vi "main.vi"() -> ()   [LabVIEW 2019]
uses:
  typedefs/basic_configuration_cluster.ctl
  typedefs/test_configuration_cluster.ctl
  typedefs/states.ctl
  typedefs/converter_configuration_cluster.ctl
  typedefs/log_data_cluster.ctl
  typedefs/operation.ctl
  typedefs/command.ctl
  <vilib>/Instr/_visa.llb/VISA Configure Serial Port (Instr).vi
panel:
  out "Configuration":T1(tab)
  in  "Ready":bool
  in  "Virtual COM port":refnum<visa-resource-name>="COM12"
  in  "Write":bool
  in  "Read":bool
  in  "data to write":T2={"version"=1, "const. voltage (mV)"=4200, "end-of-postdischarge (mAh)"=1750, "end-of-discharge (mV)"=2500, "end-of-precharge (mA or mV)"=100, "end-of-charge (mA or mV)"=100, "capacity (mAh)"=3500, "const. current char (mA)"=1750, "const. current disc (mA)"=3500} {"version" items=["Li-Ion"=1, "Ni-MH"=2]}
  out "received data":T2={"version"=1, "const. voltage (mV)"=0, "end-of-postdischarge (mAh)"=1750, "end-of-discharge (mV)"=2500, "end-of-precharge (mA or mV)"=100, "end-of-charge (mA or mV)"=100, "capacity (mAh)"=3500, "const. current char (mA)"=3500, "const. current disc (mA)"=0} {"version" items=["Li-Ion"=1, "Ni-MH"=2]}
  out "Sent":string
  out "Received":string
  out "Reception errors":string
  in  "to converter configuration":bool
  out "received data":T3={"number of cells"=1, "number of states "=8, "number of repetitions"=1, "end wait time (s)"=1200, "wait time (s)"=600, "1st state"=5, "2nd state"=11, "3rd state"=7, "4th state"=11, "5th state"=3, "6th state"=11, "7th state"=9, "8th state"=11, "9th state"=0, "10th state"=0} {"10th state" items=["not defined"=0, "charge"=3, "precharge"=5, "discharge"=7, "postdischarge"=9, "DC Resistance"=11]; "9th state" items=["not defined"=0, "charge"=3, "precharge"=5, "discharge"=7, "postdischarge"=9, "DC Resistance"=11]; "8th state" items=["not defined"=0, "charge"=3, "precharge"=5, "discharge"=7, "postdischarge"=9, "DC Resistance"=11]; "7th state" items=["not defined"=0, "charge"=3, "precharge"=5, "discharge"=7, "postdischarge"=9, "DC Resistance"=11]; "6th state" items=["not defined"=0, "charge"=3, "precharge"=5, "discharge"=7, "postdischarge"=9, "DC Resistance"=11]; "5th state" items=["not defined"=0, "charge"=3, "precharge"=5, "discharge"=7, "postdischarge"=9, "DC Resistance"=11]; "4th state" items=["not defined"=0, "charge"=3, "precharge"=5, "discharge"=7, "postdischarge"=9, "DC Resistance"=11]; "3rd state" items=["not defined"=0, "charge"=3, "precharge"=5, "discharge"=7, "postdischarge"=9, "DC Resistance"=11]; "2nd state" items=["not defined"=0, "charge"=3, "precharge"=5, "discharge"=7, "postdischarge"=9, "DC Resistance"=11]; "1st state" items=["not defined"=0, "charge"=3, "precharge"=5, "discharge"=7, "postdischarge"=9, "DC Resistance"=11]}
  out "Reception errors":string
  in  "Read 2":bool
  in  "Write 2":bool
  out "Sent":string
  out "Received":string
  in  "to test":bool
  in  "data to write":T3={"number of cells"=1, "number of states "=8, "number of repetitions"=1, "end wait time (s)"=1200, "wait time (s)"=600, "1st state"=5, "2nd state"=11, "3rd state"=7, "4th state"=11, "5th state"=3, "6th state"=11, "7th state"=9, "8th state"=11, "9th state"=0, "10th state"=0} {"10th state" items=["not defined"=0, "charge"=3, "precharge"=5, "discharge"=7, "postdischarge"=9, "DC Resistance"=11]; "9th state" items=["not defined"=0, "charge"=3, "precharge"=5, "discharge"=7, "postdischarge"=9, "DC Resistance"=11]; "8th state" items=["not defined"=0, "charge"=3, "precharge"=5, "discharge"=7, "postdischarge"=9, "DC Resistance"=11]; "7th state" items=["not defined"=0, "charge"=3, "precharge"=5, "discharge"=7, "postdischarge"=9, "DC Resistance"=11]; "6th state" items=["not defined"=0, "charge"=3, "precharge"=5, "discharge"=7, "postdischarge"=9, "DC Resistance"=11]; "5th state" items=["not defined"=0, "charge"=3, "precharge"=5, "discharge"=7, "postdischarge"=9, "DC Resistance"=11]; "4th state" items=["not defined"=0, "charge"=3, "precharge"=5, "discharge"=7, "postdischarge"=9, "DC Resistance"=11]; "3rd state" items=["not defined"=0, "charge"=3, "precharge"=5, "discharge"=7, "postdischarge"=9, "DC Resistance"=11]; "2nd state" items=["not defined"=0, "charge"=3, "precharge"=5, "discharge"=7, "postdischarge"=9, "DC Resistance"=11]; "1st state" items=["not defined"=0, "charge"=3, "precharge"=5, "discharge"=7, "postdischarge"=9, "DC Resistance"=11]}
  in  "converter configuration cluster":T5={"CVKp (x1E-3)"=1, "CVKi (x1E-3)"=8, "CVKd (x1E-1)"=1, "CCKi (x1E-3)"=1200, "CCKp (x1E-3)"=600}
  in  "Write 3":bool
  in  "Read 3":bool
  in  "to test 2":bool
  out "Received":string
  out "Sent":string
  out "Reception errors":string
  out "received data":T5={"CVKp (x1E-3)"=1, "CVKi (x1E-3)"=8, "CVKd (x1E-1)"=1, "CCKi (x1E-3)"=1200, "CCKp (x1E-3)"=600}
  out "Temperature":T6(graph)
  out "Test graph":T7(graph)
  in  "reset":bool
  in  "start":bool
  in  "next cell":bool
  in  "next state":bool
  out "log data cluster":T8={"cell counter"=1, "repetition counter"=8, "state"=1, "elapsed time (s)"=600, "voltage (mV)"=1200, "current (mA)"=1200, "capacity (mAh)"=1200, "temperature (x10E-2°C)"=1200, "duty cycle (x10E-3)"=1200}
  out "tests":bool
  out "current state":T4=1 items=["not defined"=0, "stand by"=1, "charge"=3, "precharge"=5, "discharge"=7, "postdischarge"=9, "DC Resistance"=11, "wait"=13]
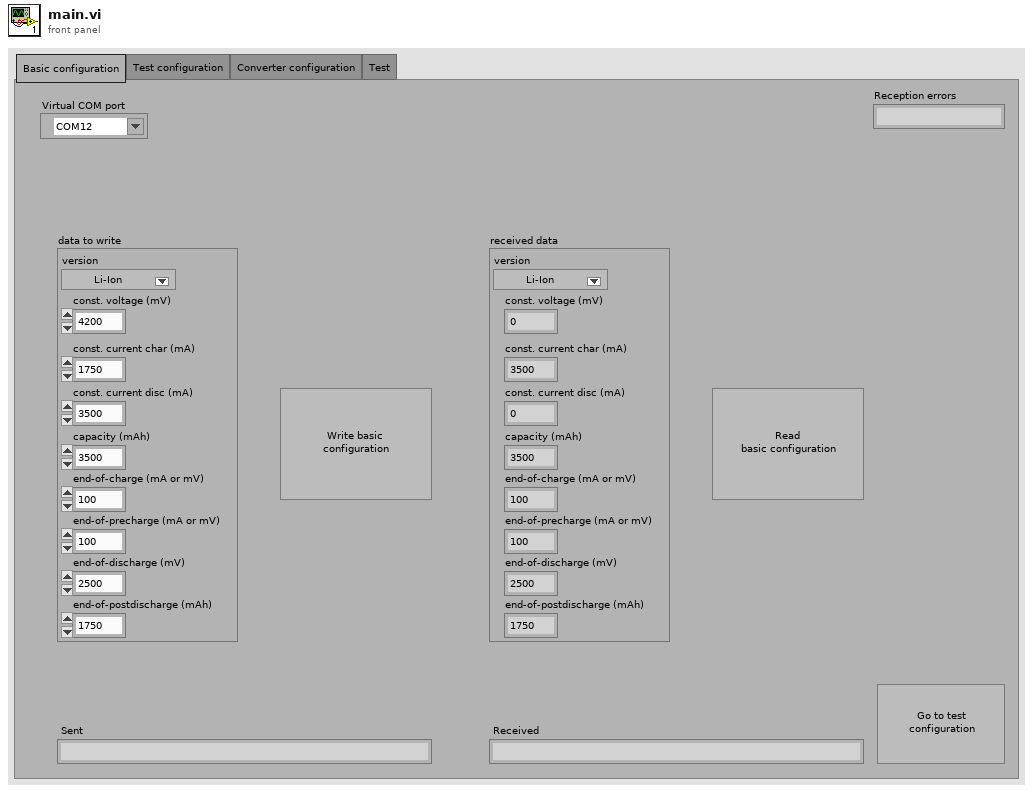
[diagram p1: front panel]
types:
  T1 = enum32{"Basic configuration", "Test configuration", "Converter configuration", "Test"}
  T2 = typedef "basic_configuration_cluster.ctl" = cluster{"version":u8, "const. voltage (mV)":u16, "end-of-postdischarge (mAh)":u16, "end-of-discharge (mV)":u16, "end-of-precharge (mA or mV)":u16, "end-of-charge (mA or mV)":u16, "capacity (mAh)":u16, "const. current char (mA)":u16, "const. current disc (mA)":u16}
  T3 = typedef "test_configuration_cluster.ctl" = cluster{"number of cells":u8, "number of states ":u8, "number of repetitions":u8, "end wait time (s)":u16, "wait time (s)":u16, "1st state":T4, "2nd state":T4, "3rd state":T4, "4th state":T4, "5th state":T4, "6th state":T4, "7th state":T4, "8th state":T4, "9th state":T4, "10th state":T4}
  T4 = typedef "states.ctl" = u8
  T5 = typedef "converter_configuration_cluster.ctl" = cluster{"CVKp (x1E-3)":u16, "CVKi (x1E-3)":u16, "CVKd (x1E-1)":u16, "CCKi (x1E-3)":u16, "CCKp (x1E-3)":u16}
  T6 = cluster{"elapsed time (s)":u16, "voltage (mV)":u16}[]
  T7 = cluster{cluster{"elapsed time (s)":u16, "capacity (mAh)":u16}[]}[]
  T8 = typedef "log_data_cluster.ctl" = cluster{"cell counter":u8, "repetition counter":u8, "state":u8, "elapsed time (s)":u16, "voltage (mV)":u16, "current (mA)":u16, "capacity (mAh)":u16, "temperature (x10E-2°C)":u16, "duty cycle (x10E-3)":u16}
  T9 = typedef "operation.ctl" = enum16{"wait", "read", "write", "action"}
  T10 = enum16{"big-endian, network order", "native, host order", "little-endian"}
  T11 = typedef "command.ctl" = enum16{"basic configuration", "test configuration", "converter configuration", "reset", "start", "next cell", "next state"}
  T12 = cluster{"elapsed time (s)":u16, "temperature (x10E-2°C)":u16}
  T13 = cluster{"elapsed time (s)":u16, "current (mA)":u16}
  T14 = cluster{"elapsed time (s)":u16, "capacity (mAh)":u16}
  T15 = cluster{"elapsed time (s)":u16, "voltage (mV)":u16}
  T16 = cluster{cluster{"elapsed time (s)":u16, "voltage (mV)":u16}[]}
  T17 = cluster{cluster{"elapsed time (s)":u16, "voltage (mV)":u16}[]}[]
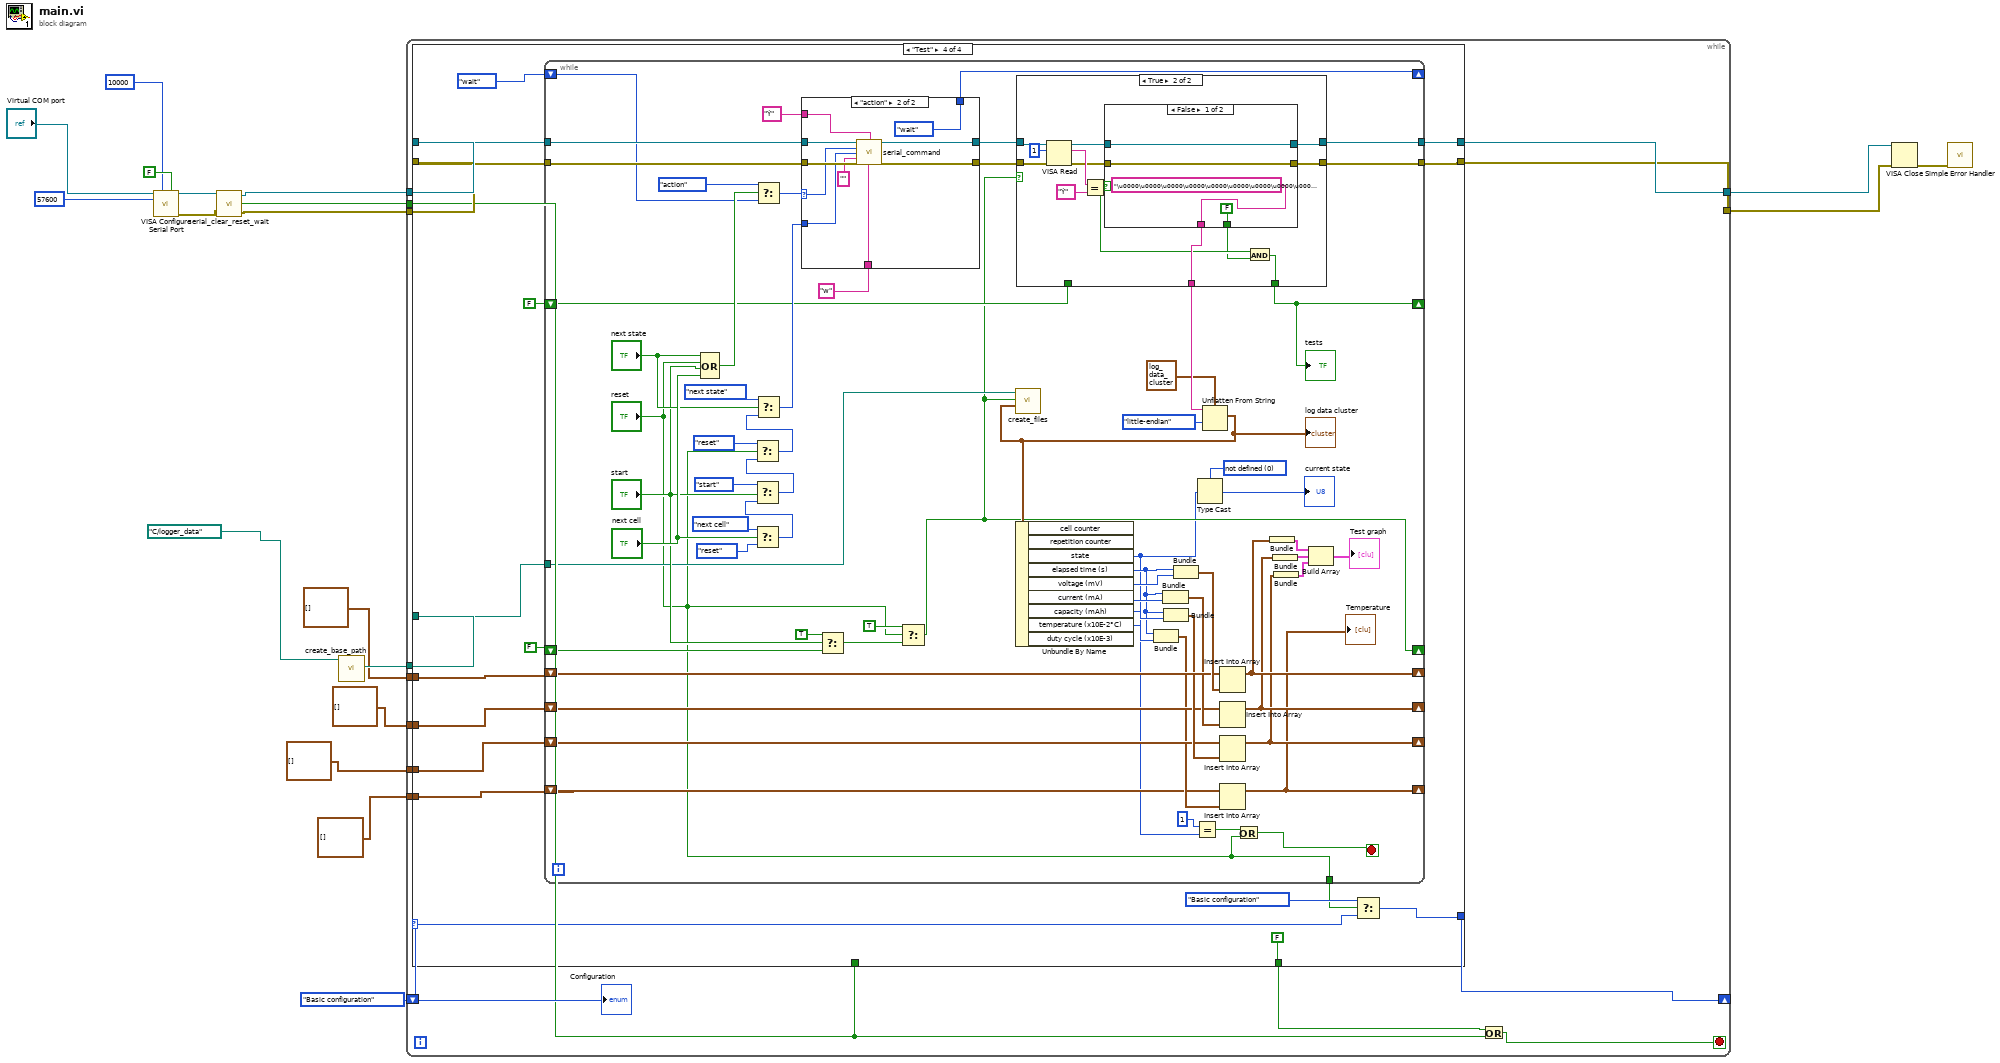
[diagram p0: block diagram]
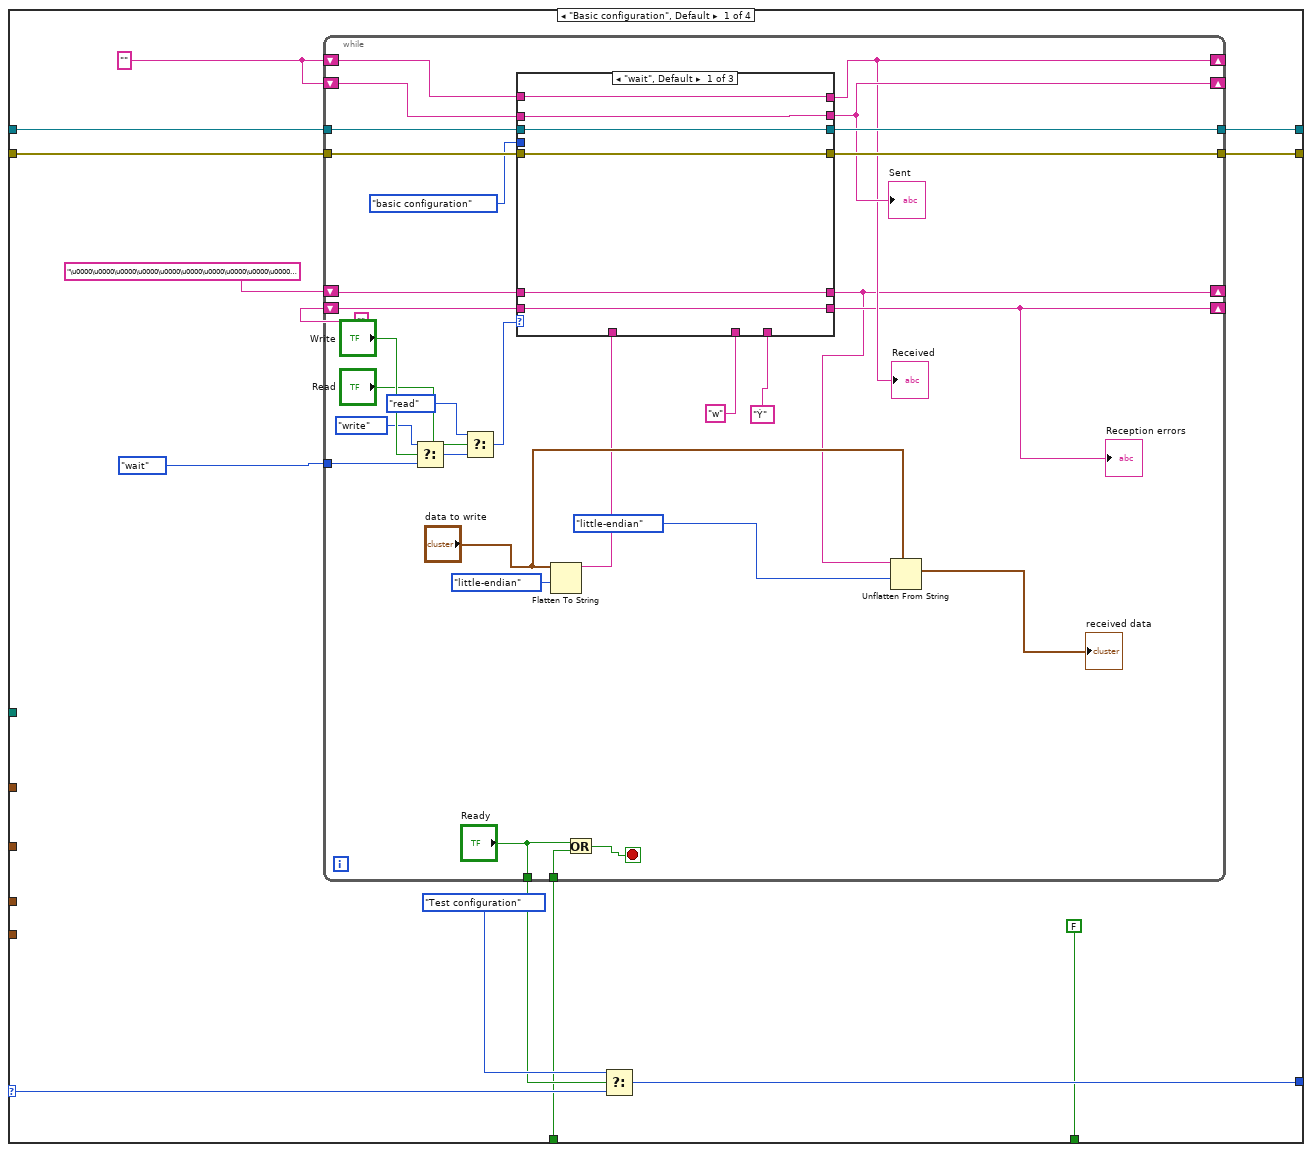
[diagram p2: hidden frame]
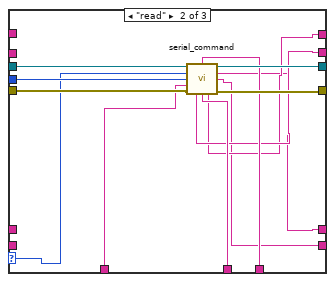
[diagram p3: hidden frame]
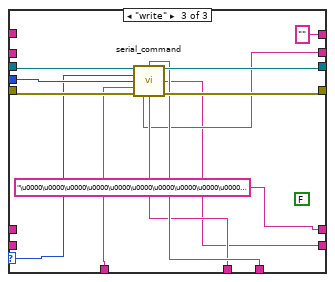
[diagram p4: hidden frame]
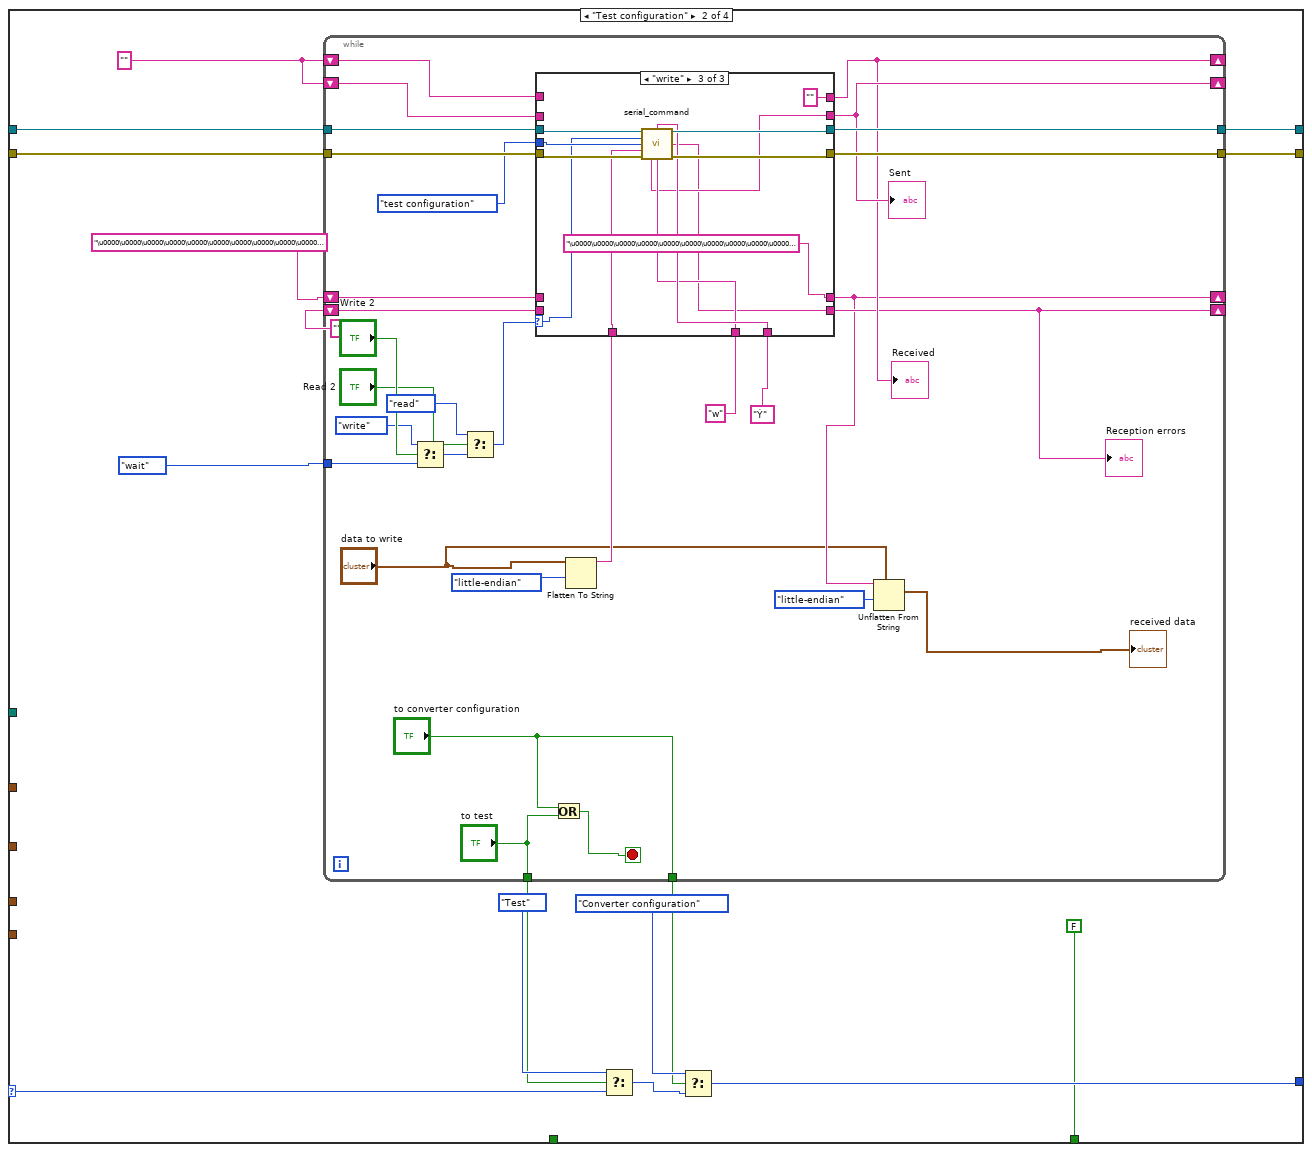
[diagram p5: hidden frame]
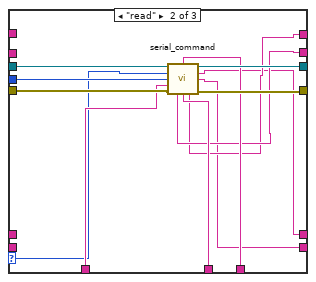
[diagram p7: hidden frame]
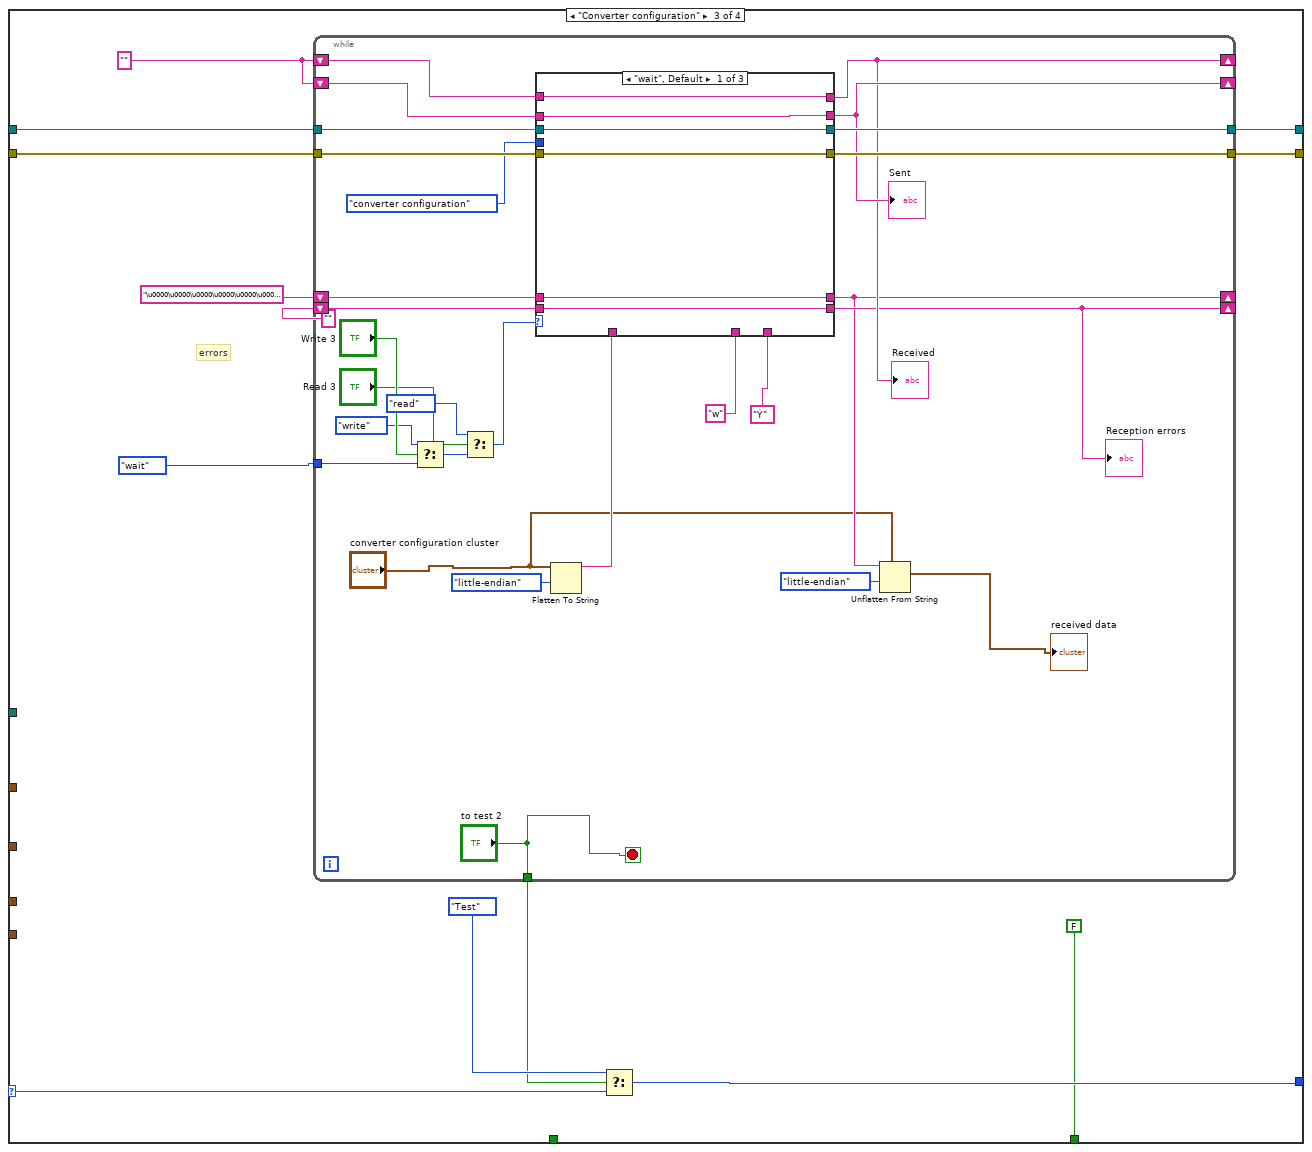
[diagram p8: hidden frame]
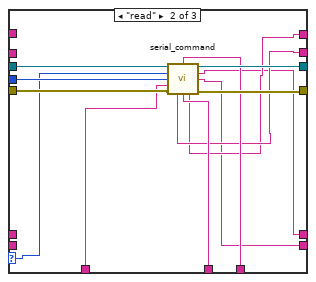
[diagram p9: hidden frame]
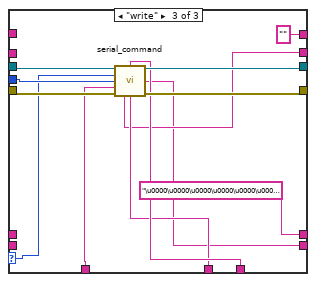
[diagram p10: hidden frame]
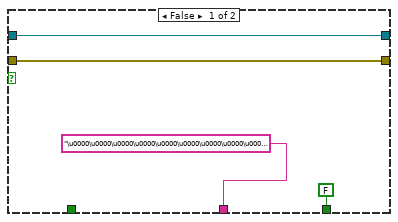
[diagram p11: hidden frame]
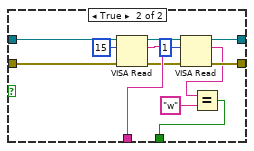
[diagram p12: hidden frame]
diagram:
  n1 = call-poly "VISA Configure Serial Port"("VISA resource name"="Virtual COM port", "timeout (10sec)"=u32 10000, "Enable Termination\nChar (T)"=FALSE ("Enable Termination\nChar (T)"), "baud rate (9600)"=u32 57600) -> ("VISA resource name out"=w17:refnum<visa-resource-name>, "error out"=w16:errorcluster)  [unwired: 10 in]
  n2 = call "serial_clear_reset_wait.vi"("VISA Refnum in"=w17, "error in (no error)"=w16) -> ("VISA Refnum out"=w12:refnum<visa-resource-name>, "test"=w8:bool, "error out"=w11:errorcluster)
  n3 = call "create_base_path.vi"("folder"=path "C:/logger_data") -> ("appended path"=w10:path)  [unwired: 10 in]
  n4 = while {
    shift-right: [w33] -> _
    shift-left: T1."Basic configuration" ("Configuration") -> [w29]
    tunnel: w12 -> [w32]
    tunnel: w11 -> [w26]
    tunnel: [w31] -> w7
    tunnel: [w30] -> w6
    tunnel: w10 -> [w28]
    tunnel: w8 -> [w25]
    tunnel: T6 [] -> [w24]
    tunnel: T6 [] -> [w23]
    tunnel: T6 [] -> [w22]
    tunnel: T6 [] -> [w21]
    stop <- w27 stop-if-true
    n5 = case shown="\"Test\"" w29 {
      selector: w29 -> [w47 w125 w200 w262]
      tunnel: [w46 w113 w191 w261] -> w33
      tunnel: w32 -> [w43 w122 w197 w276]
      tunnel: w26 -> [w42 w121 w196 w275]
      tunnel: [w41 w120 w195 w274] -> w31
      tunnel: [w40 w119 w194 w273] -> w30
      tunnel: [FALSE ("reset") FALSE ("reset") FALSE ("reset") FALSE ("reset")] -> w20
      tunnel: w28 -> [_ _ _ w270]
      tunnel: w25 -> [w34 _ _ _]
      tunnel: w24 -> [_ _ _ w269]
      tunnel: w23 -> [_ _ _ w268]
      tunnel: w22 -> [_ _ _ w267]
      tunnel: w21 -> [_ _ _ w266]
      frame "Basic configuration", Default {
        w38 = ""
        n6 = while {
          tunnel: ["Ready"] -> w44
          tunnel: w43 -> [w77]
          tunnel: w42 -> [w75]
          tunnel: [w76] -> w41
          tunnel: [w74] -> w40
          tunnel: operation."wait" -> [w73]
          shift-right: [w66] -> _
          shift-left: w38 -> [w65]
          shift-right: [w60] -> _
          shift-left: w38 -> [w64]
          shift-right: [w58] -> _
          shift-left: "" -> [w59]
          shift-right: [w53] -> _
          shift-left: "\u0000\u0000\u0000\u0000\u0000\u0000\u0000\u0000\u0000\u0000\u0000\u0000\u0000\u0000\u0000\u0000\u0000" ("data string") -> [w51]
          tunnel: w34 -> [w48]
          stop <- w50 stop-if-true
          n7 = Select(t=operation."write", s="Write", f=w73) -> (s? t:f=w70:T9)
          n8 = Select(t=operation."read", s="Read", f=w70) -> (s? t:f=w69:T9)
          n9 = Flatten To String(anything="data to write", byte order (0:big-endian, network order)=T10."little-endian") -> (data string=w52:string)  [unwired: 2 in, 2 out]
          n10 = case shown="\"wait\", Default" w69 {
            selector: w69 -> [_ w86 w99]
            tunnel: w77 -> [w83 w96 w109]
            tunnel: [w83 w94 w106] -> w76
            tunnel: w75 -> [w82 w95 w108]
            tunnel: [w82 w93 w105] -> w74
            tunnel: [w81 w90 w101] -> w66
            tunnel: w65 -> [w81 _ _]
            tunnel: [w80 w89 "" ("disassembled command")] -> w60
            tunnel: w64 -> [w80 _ _]
            tunnel: w52 -> [_ w87 w102]
            tunnel: "w" ("stop byte") -> [_ w92 w103]
            tunnel: "Ý" ("start byte") -> [_ w91 w104]
            tunnel: command."basic configuration" ("command code enum") -> [_ w88 w107]
            tunnel: w59 -> [w79 _ _]
            tunnel: [w79 w85 w97] -> w58
            tunnel: w51 -> [w78 _ _]
            tunnel: [w78 w84 "\u0000\u0000\u0000\u0000\u0000\u0000\u0000\u0000\u0000\u0000\u0000\u0000\u0000\u0000\u0000\u0000\u0000" ("data string")] -> w53
            frame "wait", Default {
            }
            frame "read" {
              n11 = call "serial_command.vi"("VISA in"=w96, "start byte"=w91, "operation enum"=w86, "command code enum"=w88, "data"=w87, "error in"=w95, "stop byte"=w92) -> ("VISA out"=w94:refnum<visa-resource-name>, "data"=w84:string, "error"=w85:string, "assembled command"=w90:string, "disassembled command"=w89:string, "error out"=w93:errorcluster)  [unwired: 1 in, 2 out]
            }
            frame "write" {
              (unwired) FALSE ("tests")
              n12 = call "serial_command.vi"("VISA in"=w109, "start byte"=w104, "operation enum"=w99, "command code enum"=w107, "data"=w102, "error in"=w108, "stop byte"=w103) -> ("VISA out"=w106:refnum<visa-resource-name>, "error"=w97:string, "assembled command"=w101:string, "error out"=w105:errorcluster)  [unwired: 1 in, 4 out]
            }
          }
          "Sent" <- w66
          "Received" <- w60
          "Reception errors" <- w58
          n13 = Or(x="Ready", y=w48) -> (x .or. y?=w50:bool)
          n14 = Unflatten From String(type="data to write", binary string=w53, byte order (0:big-endian, network order)=T10."little-endian") -> (value=→"received data":T2)  [unwired: 2 in, 2 out]
        }
        n15 = Select(t=T1."Test configuration", s=w44, f=w47) -> (s? t:f=w46:T1)
      }
      frame "Test configuration" {
        w117 = ""
        n16 = while {
          tunnel: ["to test"] -> w123
          tunnel: w122 -> [w155]
          tunnel: w121 -> [w153]
          tunnel: [w154] -> w120
          tunnel: [w152] -> w119
          tunnel: operation."wait" -> [w151]
          shift-right: [w144] -> _
          shift-left: w117 -> [w143]
          shift-right: [w137] -> _
          shift-left: w117 -> [w142]
          tunnel: ["to converter configuration"] -> w114
          shift-right: [w132] -> _
          shift-left: "" -> [w133]
          shift-right: [w130] -> _
          shift-left: "\u0000\u0000\u0000\u0000\u0000\u0000\u0000\u0000\u0000\u0000\u0000\u0000\u0000\u0000\u0000\u0000\u0000" ("data string") -> [w127]
          stop <- w134 stop-if-true
          n17 = Select(t=operation."write", s="Write 2", f=w151) -> (s? t:f=w148:T9)
          n18 = Select(t=operation."read", s="Read 2", f=w148) -> (s? t:f=w147:T9)
          n19 = Or(x="to converter configuration", y="to test") -> (x .or. y?=w134:bool)
          n20 = Flatten To String(anything="data to write", byte order (0:big-endian, network order)=T10."little-endian") -> (data string=w141:string)  [unwired: 2 in, 2 out]
          n21 = case shown="\"write\"" w147 {
            selector: w147 -> [_ w163 w177]
            tunnel: w155 -> [w161 w174 w187]
            tunnel: [w161 w172 w184] -> w154
            tunnel: w153 -> [w160 w173 w186]
            tunnel: [w160 w171 w183] -> w152
            tunnel: [w159 w168 w179] -> w144
            tunnel: w143 -> [w159 _ _]
            tunnel: [w158 w167 "" ("disassembled command")] -> w137
            tunnel: w142 -> [w158 _ _]
            tunnel: w141 -> [_ w164 w180]
            tunnel: "w" ("stop byte") -> [_ w170 w181]
            tunnel: "Ý" ("start byte") -> [_ w169 w182]
            tunnel: [w156 w166 "\u0000\u0000\u0000\u0000\u0000\u0000\u0000\u0000\u0000\u0000\u0000\u0000\u0000\u0000\u0000\u0000\u0000" ("data string")] -> w130
            tunnel: command."test configuration" ("command code enum") -> [_ w165 w185]
            tunnel: [w157 w162 w175] -> w132
            tunnel: w133 -> [w157 _ _]
            tunnel: w127 -> [w156 _ _]
            frame "wait", Default {
            }
            frame "read" {
              n22 = call "serial_command.vi"("VISA in"=w174, "start byte"=w169, "operation enum"=w163, "command code enum"=w165, "data"=w164, "error in"=w173, "stop byte"=w170) -> ("VISA out"=w172:refnum<visa-resource-name>, "data"=w166:string, "error"=w162:string, "assembled command"=w168:string, "disassembled command"=w167:string, "error out"=w171:errorcluster)  [unwired: 1 in, 2 out]
            }
            frame "write" {
              n23 = call "serial_command.vi"("VISA in"=w187, "start byte"=w182, "operation enum"=w177, "command code enum"=w185, "data"=w180, "error in"=w186, "stop byte"=w181) -> ("VISA out"=w184:refnum<visa-resource-name>, "error"=w175:string, "assembled command"=w179:string, "error out"=w183:errorcluster)  [unwired: 1 in, 4 out]
            }
          }
          "Sent" <- w144
          "Received" <- w137
          "Reception errors" <- w132
          n24 = Unflatten From String(type="data to write", binary string=w130, byte order (0:big-endian, network order)=T10."little-endian") -> (value=→"received data":T3)  [unwired: 2 in, 2 out]
        }
        n25 = Select(t=T1."Test", s=w123, f=w125) -> (s? t:f=w116:T1)
        n26 = Select(t=T1."Converter configuration", s=w114, f=w116) -> (s? t:f=w113:T1)
      }
      frame "Converter configuration" {
        w192 = ""
        # "errors"
        n27 = while {
          tunnel: ["to test 2"] -> w198
          tunnel: w197 -> [w228]
          tunnel: w196 -> [w226]
          tunnel: [w227] -> w195
          tunnel: [w225] -> w194
          tunnel: operation."wait" -> [w224]
          shift-right: [w217] -> _
          shift-left: w192 -> [w216]
          shift-right: [w210] -> _
          shift-left: w192 -> [w215]
          shift-right: [w207] -> _
          shift-left: "" -> [w208]
          shift-right: [w204] -> _
          shift-left: "\u0000\u0000\u0000\u0000\u0000\u0000\u0000\u0000\u0000\u0000" ("data string") -> [w205]
          stop <- "to test 2" stop-if-true
          n28 = Select(t=operation."write", s="Write 3", f=w224) -> (s? t:f=w221:T9)
          n29 = Select(t=operation."read", s="Read 3", f=w221) -> (s? t:f=w220:T9)
          n30 = Flatten To String(anything="converter configuration cluster", byte order (0:big-endian, network order)=T10."little-endian") -> (data string=w214:string)  [unwired: 2 in, 2 out]
          n31 = case shown="\"wait\", Default" w220 {
            selector: w220 -> [_ w236 w250]
            tunnel: w228 -> [w234 w247 w260]
            tunnel: [w234 w245 w257] -> w227
            tunnel: w226 -> [w233 w246 w259]
            tunnel: [w233 w244 w256] -> w225
            tunnel: [w232 w241 w252] -> w217
            tunnel: w216 -> [w232 _ _]
            tunnel: [w231 w240 "" ("disassembled command")] -> w210
            tunnel: w215 -> [w231 _ _]
            tunnel: w214 -> [_ w237 w253]
            tunnel: "w" ("stop byte") -> [_ w243 w254]
            tunnel: "Ý" ("start byte") -> [_ w242 w255]
            tunnel: [w229 w239 "\u0000\u0000\u0000\u0000\u0000\u0000\u0000\u0000\u0000\u0000" ("data string")] -> w204
            tunnel: command."converter configuration" ("command code enum") -> [_ w238 w258]
            tunnel: w208 -> [w230 _ _]
            tunnel: [w230 w235 w248] -> w207
            tunnel: w205 -> [w229 _ _]
            frame "wait", Default {
            }
            frame "read" {
              n32 = call "serial_command.vi"("VISA in"=w247, "start byte"=w242, "operation enum"=w236, "command code enum"=w238, "data"=w237, "error in"=w246, "stop byte"=w243) -> ("VISA out"=w245:refnum<visa-resource-name>, "data"=w239:string, "error"=w235:string, "assembled command"=w241:string, "disassembled command"=w240:string, "error out"=w244:errorcluster)  [unwired: 1 in, 2 out]
            }
            frame "write" {
              n33 = call "serial_command.vi"("VISA in"=w260, "start byte"=w255, "operation enum"=w250, "command code enum"=w258, "data"=w253, "error in"=w259, "stop byte"=w254) -> ("VISA out"=w257:refnum<visa-resource-name>, "error"=w248:string, "assembled command"=w252:string, "error out"=w256:errorcluster)  [unwired: 1 in, 4 out]
            }
          }
          "Sent" <- w217
          "Received" <- w210
          "Reception errors" <- w207
          n34 = Unflatten From String(type="converter configuration cluster", binary string=w204, byte order (0:big-endian, network order)=T10."little-endian") -> (value=→"received data":T5)  [unwired: 2 in, 2 out]
        }
        n35 = Select(t=T1."Test", s=w198, f=w200) -> (s? t:f=w191:T1)
      }
      frame "Test" {
        n36 = while {
          tunnel: w276 -> [w331]
          tunnel: w275 -> [w330]
          tunnel: [w324] -> w274
          tunnel: [w326] -> w273
          shift-right: [w290] -> _
          shift-left: FALSE -> [w320]
          shift-right: [w314] -> _
          shift-left: FALSE -> [w315]
          shift-right: [w309] -> _
          shift-left: operation."wait" ("Enum") -> [w311]
          shift-right: [w297] -> _
          shift-left: w267 -> [w301]
          shift-right: [w299] -> _
          shift-left: w269 -> [w305]
          shift-right: [w298] -> _
          shift-left: w268 -> [w300]
          tunnel: w270 -> [w291]
          shift-right: [w285] -> _
          shift-left: w266 -> [w286]
          tunnel: ["reset"] -> w263
          stop <- w279 stop-if-true
          w284 = T4 0 items=["not defined"=0, "stand by"=1, "charge"=3, "precharge"=5, "discharge"=7, "postdischarge"=9, "DC Resistance"=11] ("1st state")
          n37 = Compound Arithmetic op=OR("next state", "reset", "start", "next cell") -> (w322:bool)
          n38 = Select(t=command."next cell", s="next cell", f=command."reset" ("command code enum")) -> (s? t:f=w338:T11)
          n39 = Select(t=command."start", s="start", f=w338) -> (s? t:f=w336:T11)
          n40 = Select(t=command."reset", s="reset", f=w336) -> (s? t:f=w334:T11)
          n41 = Select(t=operation."action" ("Enum"), s=w322, f=w311) -> (s? t:f=w310:T9)
          n42 = Select(t=command."next state", s="next state", f=w334) -> (s? t:f=w321:T11)
          n43 = case shown="\"action\"" w310 {
            selector: w310 -> [w376 w384]
            tunnel: w321 -> [_ w383]
            tunnel: w331 -> [w377 w388]
            tunnel: w330 -> [w378 w387]
            tunnel: [w377 w386] -> w325
            tunnel: [w378 w385] -> w327
            tunnel: "Ý" ("start byte") -> [_ w380]
            tunnel: "w" ("stop byte") -> [_ w381]
            tunnel: [w376 operation."wait" ("Enum")] -> w309
            frame "wait", Default {
            }
            frame "action" {
              n44 = call "serial_command.vi"("VISA in"=w388, "start byte"=w380, "operation enum"=w384, "command code enum"=w383, "data"="", "error in"=w387, "stop byte"=w381) -> ("VISA out"=w386:refnum<visa-resource-name>, "error out"=w385:errorcluster)  [unwired: 1 in, 6 out]
            }
          }
          n45 = Select(t=TRUE, s="start", f=w320) -> (s? t:f=w317:bool)
          n46 = Select(t=TRUE, s="reset", f=w317) -> (s? t:f=w290:bool)
          n47 = case shown="True" w290 {
            tunnel: w327 -> [w344 w359]
            tunnel: [w344 w350] -> w326
            tunnel: w325 -> [w345 w358]
            tunnel: [w345 w351] -> w324
            tunnel: ["\u0000\u0000\u0000\u0000\u0000\u0000\u0000\u0000\u0000\u0000\u0000\u0000\u0000\u0000\u0000" ("read buffer 2") w352] -> w323
            tunnel: [FALSE w347] -> w314
            tunnel: w315 -> [_ _]
            frame False {
            }
            frame True {
              n48 = VISA Read(VISA resource name=w358, byte count=u32 1, error in (no error)=w359) -> (VISA resource name out=w354:refnum<visa-resource-name>, read buffer=w356:string, error out=w353:errorcluster)  [unwired: 1 out]
              n49 = Equal?(x=w356, y="Ý") -> (x = y?=w349:bool)
              n50 = case shown="False" w349 {
                tunnel: w354 -> [w362 w374]
                tunnel: w353 -> [w361 w375]
                tunnel: ["\u0000\u0000\u0000\u0000\u0000\u0000\u0000\u0000\u0000\u0000\u0000\u0000\u0000\u0000\u0000" ("read buffer 2") w373] -> w352
                tunnel: [w362 w368] -> w351
                tunnel: [w361 w367] -> w350
                tunnel: [FALSE w364] -> w348
                frame False {
                }
                frame True {
                  n51 = VISA Read(VISA resource name=w374, byte count=u32 15, error in (no error)=w375) -> (VISA resource name out=w371:refnum<visa-resource-name>, read buffer=w373:string, error out=w370:errorcluster)  [unwired: 1 out]
                  n52 = VISA Read(VISA resource name=w371, byte count=u32 1, error in (no error)=w370) -> (VISA resource name out=w368:refnum<visa-resource-name>, read buffer=w366:string, error out=w367:errorcluster)  [unwired: 1 out]
                  n53 = Equal?(x=w366, y="w") -> (x = y?=w364:bool)
                }
              }
              n54 = And(x=w349, y=w348) -> (x .and. y?=w347:bool)
            }
          }
          "tests" <- w314
          n55 = Unflatten From String(type=T8 {"cell counter"=1, "repetition counter"=8, "state"=1, "elapsed time (s)"=600, "voltage (mV)"=1200, "current (mA)"=1200, "capacity (mAh)"=1200, "temperature (x10E-2°C)"=1200, "duty cycle (x10E-3)"=1200} ("log data cluster"), binary string=w323, byte order (0:big-endian, network order)=T10."little-endian") -> (value=w292:T8)  [unwired: 2 in, 2 out]
          "log data cluster" <- w292
          n56 = call "create_files.vi"("log data cluster"=w292, "start?"=w290, "base path"=w291) -> ()  [unwired: 9 in]
          n57 = Unbundle By Name(w292) -> ("state"=w281:u8, "elapsed time (s)"=w289:u16, "voltage (mV)"=w308:u16, "current (mA)"=w307:u16, "capacity (mAh)"=w303:u16, "temperature (x10E-2°C)"=w288:u16)  [unwired: 3 out]
          n58 = Bundle("elapsed time (s)"=w289, "temperature (x10E-2°C)"=w288) -> (w287:T12)  [unwired: 1 in]
          n59 = Bundle("elapsed time (s)"=w289, "current (mA)"=w307) -> (w304:T13)  [unwired: 1 in]
          n60 = Bundle("elapsed time (s)"=w289, "capacity (mAh)"=w303) -> (w302:T14)  [unwired: 1 in]
          n61 = Bundle("elapsed time (s)"=w289, "voltage (mV)"=w308) -> (w306:T15)  [unwired: 1 in]
          n62 = Equal?(x=1, y=w281) -> (x = y?=w280:bool)
          n63 = Type Cast(type=w284, x=w281) -> (*(type *) &x=→"current state":T4)
          n64 = Insert Into Array(array=w305, new element=w306) -> (w299:T6)  [unwired: 1 in]
          n65 = Insert Into Array(array=w300, new element=w304) -> (w298:T6)  [unwired: 1 in]
          n66 = Insert Into Array(array=w301, new element=w302) -> (w297:T6)  [unwired: 1 in]
          n67 = Insert Into Array(array=w286, new element=w287) -> (w285:T6)  [unwired: 1 in]
          "Temperature" <- w285
          n68 = Or(x=w280, y="reset") -> (x .or. y?=w279:bool)
          n69 = Bundle(w299) -> (w296:T16)  [unwired: 1 in]
          n70 = Bundle(w298) -> (w295:T16)  [unwired: 1 in]
          n71 = Bundle(w297) -> (w294:T16)  [unwired: 1 in]
          n72 = Build Array(w296, w295, w294) -> (→"Test graph":T17)
        }
        n73 = Select(t=T1."Basic configuration", s=w263, f=w262) -> (s? t:f=w261:T1)
      }
    }
    n74 = Or(x=w20, y=w25) -> (x .or. y?=w27:bool)
    "Configuration" <- w29
  }
  n75 = VISA Close(VISA resource name=w7, error in (no error)=w6) -> (error out=w5:errorcluster)
  n76 = call <vilib>:"Simple Error Handler.vi"("error in (no error)"=w5) -> ()  [unwired: 4 in, 5 out]
